vi "Generate Signal.vi"() -> ()   [LabVIEW 2011, in "Simple Plugin.lvclass"]
uses:
  Simple Plugin.lvclass
  <vilib>/measure/NI_MABase.lvlib
  Parent Plugin Definition/Plugin Template/Generic Plugin.lvclass
panel:
  in  "Dial":dbl(knob) scale=0.0..10.0
  out "Waveform Graph":waveform(dbl)(graph)
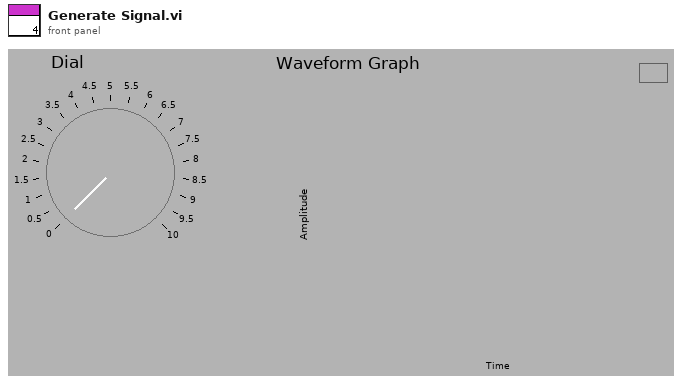
[diagram p1: front panel]
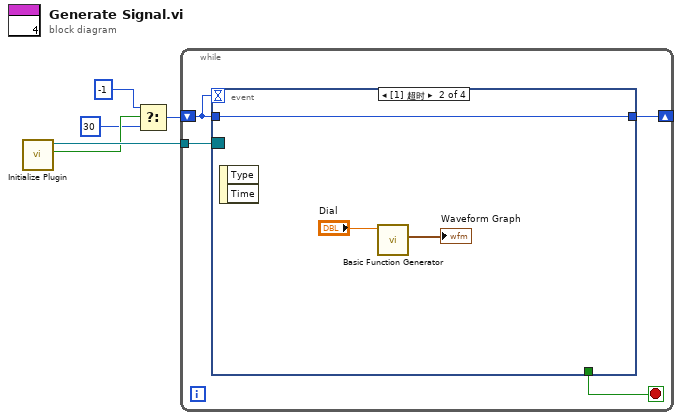
[diagram p0: block diagram]
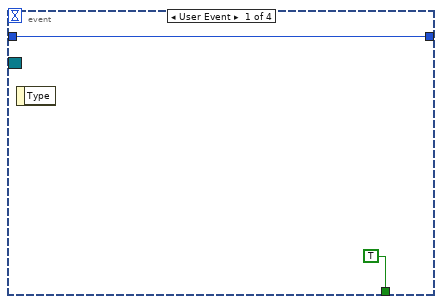
[diagram p2: hidden frame]
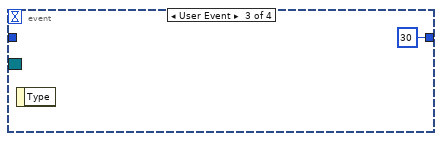
[diagram p3: hidden frame]
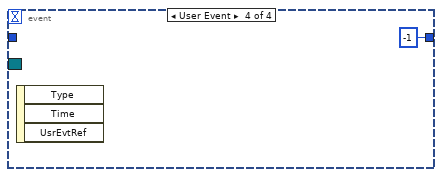
[diagram p4: hidden frame]
diagram:
  n1 = call "Initialize Plugin.vi"() -> ("Called From Framework? Yes (T) No (F)"=w3:bool, "Event Registration Refnum"=w5:refnum<event-registration>)  [unwired: 9 in, 1 out]
  n2 = Select(t=-1, s=w3, f=30) -> (s? t:f=w4:i32)
  n3 = while {
    tunnel: w5 -> [w9]
    shift-right: [w6] -> _
    shift-left: w4 -> [w7]
    stop <- w8 stop-if-true
    n4 = event shown="[1] 超时" {
      selector: w9 -> [_ _ _ _]
      dyn-events: _ -> [_ _ _ _]
      timeout: w7 -> [_ _ _ _]
      tunnel: [TRUE _ _ _] -> w8
      tunnel: w7 -> [w10 w12 _ _]
      tunnel: [w10 w12 30 -1] -> w6
      event User Event {
        n5 = event-data() -> ()  [unwired: 1 in, 1 out]
      }
      event Timeout {
        n6 = event-data() -> ()  [unwired: 1 in, 2 out]
        n7 = call <vilib>:"Basic Function Generator.vi"("frequency"="Dial") -> ("signal out"=→"Waveform Graph":waveform(dbl))  [unwired: 8 in, 2 out]
      }
      event User Event {
        n8 = event-data() -> ()  [unwired: 1 in, 1 out]
      }
      event User Event {
        n9 = event-data() -> ()  [unwired: 1 in, 3 out]
      }
    }
  }
